vi "Climb Controller.vi"(8 "error in":errorcluster) -> ()   [LabVIEW 2020]
doc: "This VI executes continuously carrying out the current operation and responding to updates or new operations. It will often contain the timing or control code that is difficult to place directly in TeleOp. This VI generally opens all sensors and motors and isolates the rest of the robot code from knowing how the operations are carried out."
uses:
  <vilib>/Rock Robotics/WPI/Framework/Completion Status.ctl
  Climb Setpoints.ctl
  Climb Operations.ctl
  <vilib>/Rock Robotics/WPI/ThirdParty/Phoenix-LabVIEW/Motor Controller/Controls/CTRE_Phoenix_MotorControl_ControlMode.ctl
  <vilib>/Rock Robotics/Network Tables/NT Write Number.vi
panel:
  in  "Interactive Values":T1
  out "Current\nCmd":string
  in  "Buttons":cluster{"Execute Cmd":bool, "Abort Cmd":bool}
  out "Command Timing":cluster{"Start Time (ms)":u32, "Iterations":i32}
  out "Status":T3
  # "Tip: It may be helpful to observe inputs and sensor values.\nYou may also want to display tuning or debugging controls."
  # "Interactive Command: You may fill in the settings for a command\nand schedule it with the Execute button. You can observe and abort\nany command while fine tuning the code for the controller."
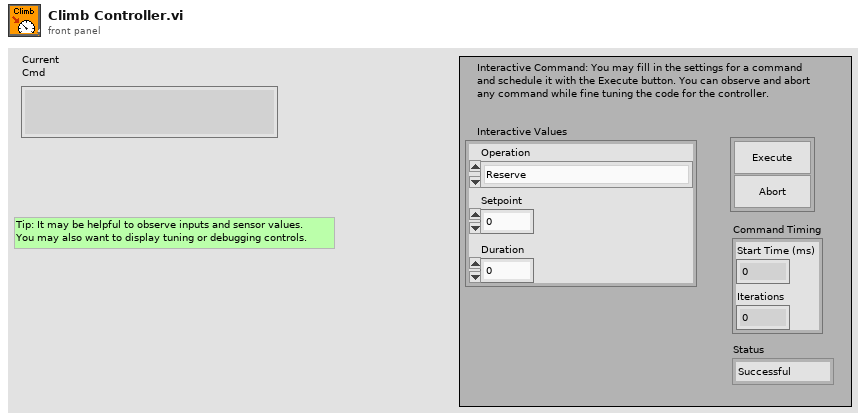
[diagram p1: front panel]
types:
  T1 = typedef "Climb Setpoints.ctl" = cluster{"Operation":T2, "Setpoint":dbl, "Duration":dbl}
  T2 = typedef "Climb Operations.ctl" = enum16{"Reserve", "Read Current", "Immediate", "Up", "Down"}
  T3 = typedef "Completion Status.ctl" = enum16{"Successful", "Aborted", "Incomplete"}
  T4 = typedef "WPI_MotorControlDeviceRef.ctl" = cluster{"DeviceStatus":errorcluster, "Type":T5, "PWM":cluster{"PWM Channel":T6, "DeadBand":T7}, "CAN":cluster{"Device Number":u8, "SetOutput VI Ref":variant, "GetOutput VI Ref":variant, "Enable VI Ref":variant, "Disable VI Ref":variant, "Data":variant}, "Invert":bool, "DIO PWM":cluster{"PWM \"Enable\" Channel":T6, "DIOChannel":T8, "PWM Rate":dbl}}
  T5 = typedef "WPI_MotorControlType.ctl" = enum16{"PWM", "CAN", "DIO PWM"}
  T6 = typedef "FPGA_DIOPWMChannel.ctl" = enum8{"PWM 0", "PWM 1", "PWM 2", "PWM 3", "PWM 4", "PWM 5", "PWM 6", "PWM 7", "PWM 8", "PWM 9", "PWM MXP 0", "PWM MXP 1", "PWM MXP 2", "PWM MXP 3", "PWM MXP 4", "PWM MXP 5", "PWM MXP 6", "PWM MXP 7", "PWM MXP 8", "PWM MXP 9", "Invalid"}
  T7 = typedef "WPI_PWMDeadband.ctl" = cluster{"Name":string, "maxPositivePwm":i32, "minPositivePwm":i32, "centerPwm":i32, "maxNegativePwm":i32, "minNegativePwm":i32, "angularRange":u16}
  T8 = typedef "FPGA_DIOChannel.ctl" = enum8{"DIO 0", "DIO 1", "DIO 2", "DIO 3", "DIO 4", "DIO 5", "DIO 6", "DIO 7", "DIO 8", "DIO 9", "DIO MXP 0", "DIO MXP 1", "DIO MXP 2", "DIO MXP 3", "DIO MXP 4", "DIO MXP 5", "DIO MXP 6", "DIO MXP 7", "DIO MXP 8", "DIO MXP 9", "DIO MXP 10", "DIO MXP 11", "DIO MXP 12", "DIO MXP 13", "DIO MXP 14", "DIO MXP 15", "SPI Port CS1", "SPI Port CS2", "SPI Port CS3", "SPI Port MISO", "SPI Port MOSI", "Invalid"}
  T9 = typedef "Command Status Info.ctl" = cluster{"Name":string, "Status":T3, "notifier out":T10}
  T10 = typedef "Completion Notifier.ctl" = refnum<notifier>
  T11 = cluster{"Current Command":T1, "Command Timing":cluster{"Start Time (ms)":u32, "Iterations":i32}, "Command Arguments":cluster{"Command Info":T9, "Description":string, "Default Command":T1, "queue out":refnum<queue>, "Subsystem Name":string}}
  T12 = typedef "CTRE_Phoenix_MotorControl_ControlMode.ctl" = u16
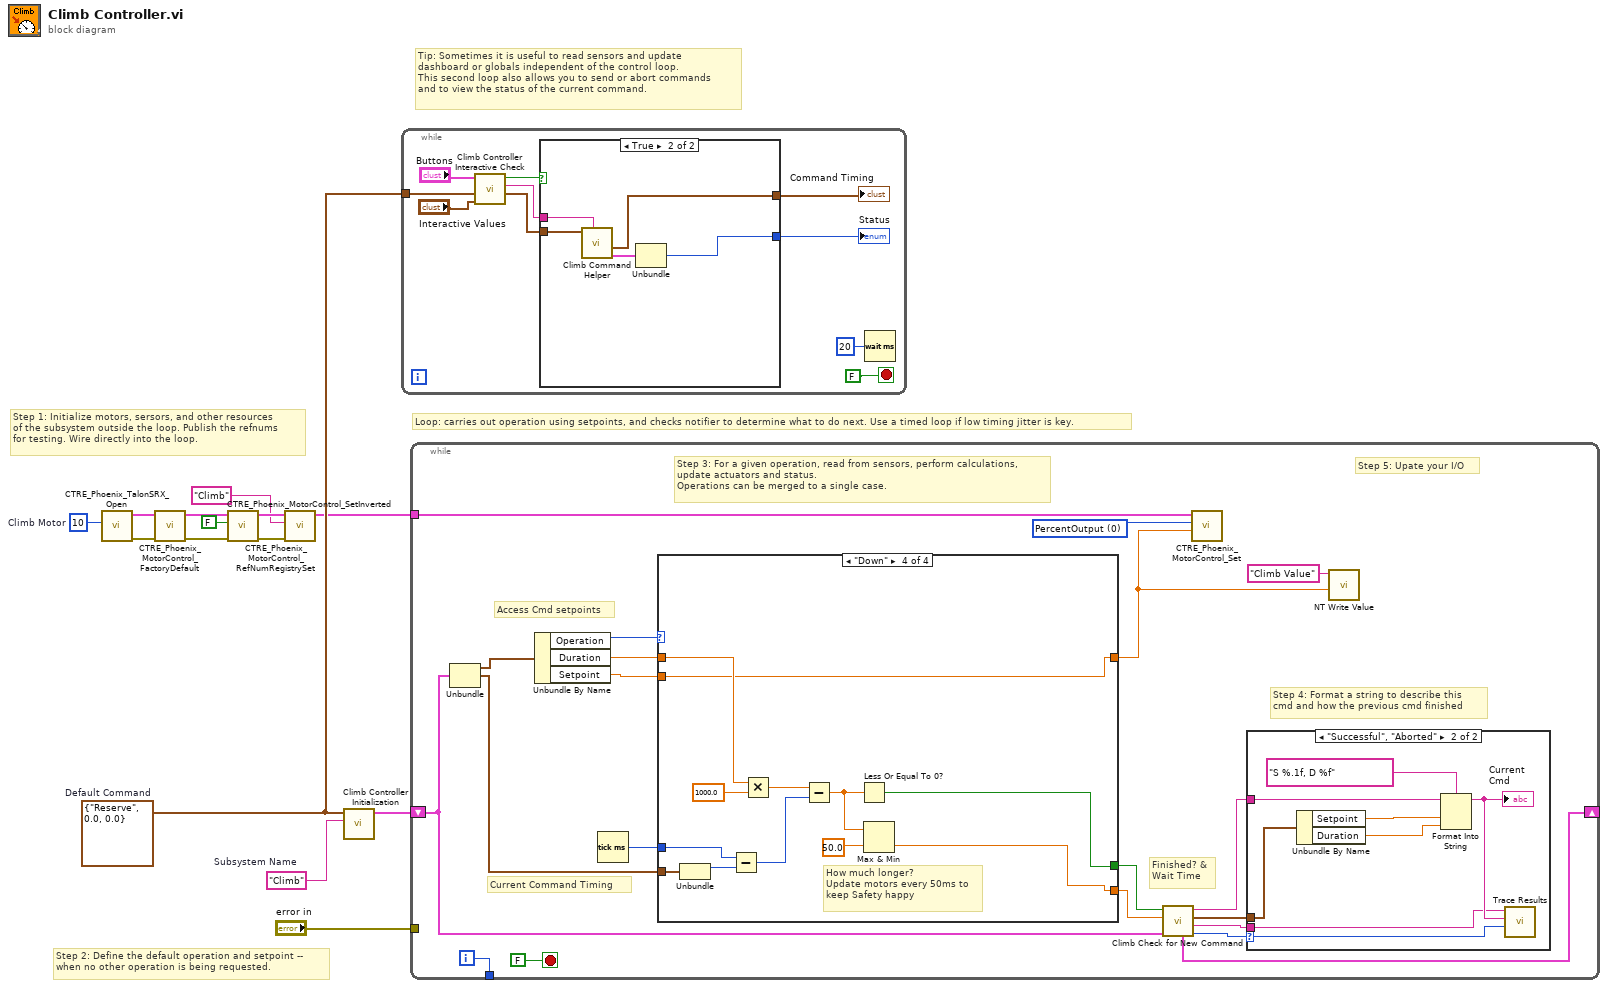
[diagram p0: block diagram]
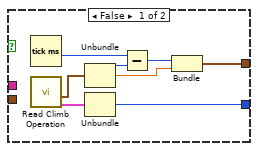
[diagram p2: hidden frame]
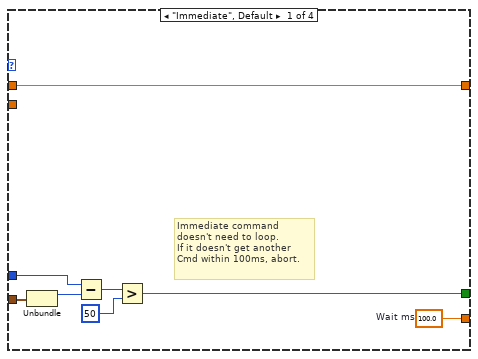
[diagram p4: hidden frame]
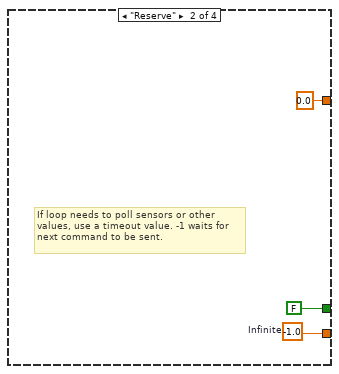
[diagram p5: hidden frame]
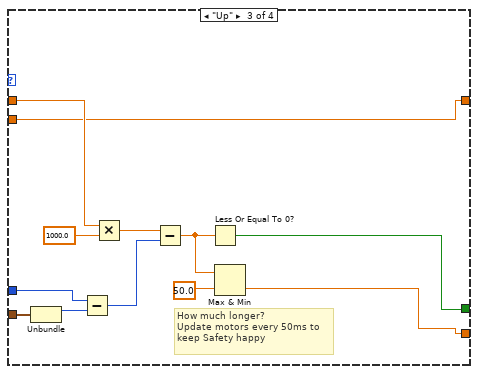
[diagram p6: hidden frame]
diagram:
  w2 = u8 10  # Climb Motor
  w11 = T1 {"Operation"=enum."Reserve", "Setpoint"=0.0, "Duration"=0.0}  # Default Command
  w12 = "Climb"  # Subsystem Name
  # "Tip: Sometimes it is useful to read sensors and update\ndashboard or globals independent of the control loop.\nThis second loop also allows you to send or abort commands\nand to view the status of the current command."
  # "Step 2: Define the default operation and setpoint --\nwhen no other operation is being requested."
  # "Step 1: Initialize motors, sersors, and other resources\nof the subsystem outside the loop. Publish the refnums\nfor testing. Wire directly into the loop."
  # "Loop: carries out operation using setpoints, and checks notifier to determine what to do next. Use a timed loop if low timing jitter is key."
  n1 = call <vilib>:"CTRE_Phoenix_TalonSRX_Open.vi"("Device Number"=w2) -> ("error out"=w10:errorcluster, "PhoenixMotorControlDevRef"=w9:T4)  [unwired: 9 in]
  n2 = call <vilib>:"CTRE_Phoenix_MotorControl_FactoryDefault.vi"("error in"=w10, "PhoenixMotorControlDevRef"=w9) -> ("error out"=w8:errorcluster, "PhoenixMotorControlDevRef"=w7:T4)  [unwired: 8 in]
  n3 = call <vilib>:"CTRE_Phoenix_MotorControl_SetInverted.vi"("error in (no error)"=w8, "Invert?"=FALSE, "PhoenixMotorControlDevRef"=w7) -> ("error out"=w6:errorcluster, "PhoenixMotorControlDevRef"=w5:T4)  [unwired: 7 in]
  n4 = call <vilib>:"CTRE_Phoenix_MotorControl_RefNumRegistrySet.vi"("error in (no error)"=w6, "refnum name"="Climb", "PhoenixMotorControlDevRef"=w5) -> ("PhoenixMotorControlDevRef"=w1:T4)  [unwired: 7 in, 1 out]
  n5 = call "Climb Controller Initialization.vi"("Subsystem Name"=w12, "Default Command"=w11) -> ("Current Command"=w13:T11)  [unwired: 9 in]
  n6 = while {
    tunnel: w11 -> [w21]
    stop <- FALSE stop-if-true
    n7 = call "Climb Controller Interactive Check.vi"("Interactive Command in"="Interactive Values", "Default Command"=w21, "Buttons"="Buttons") -> ("Interactive Command out"=w18:T1, "Trace String"=w19:string, "Schedule"=w20:bool)  [unwired: 6 in]
    n8 = case shown="True" w20 {
      tunnel: [w32 w37] -> w17
      tunnel: w18 -> [_ w35]
      tunnel: [w28 w33] -> w16
      tunnel: w19 -> [_ w36]
      frame False {
        n9 = Tick Count (ms)() -> (millisecond timer value=w27:u32)
        n10 = call "Read Climb Operation.vi"() -> ("Command Info"=w25:T9, "SubSystem Data"=w26:T1)  [unwired: 9 in, 1 out]
        n11 = Unbundle(w26) -> ("Operation"=w31:T2, "Setpoint"=w29:dbl)  [unwired: 1 out]
        n12 = Unbundle(w25) -> ("Status"=w32:T3)  [unwired: 2 out]
        n13 = Subtract(x=w27, y=w31) -> (x-y=w30:u32)
        n14 = Bundle(w30, "Setpoint"=w29) -> (w28:cluster{u32, "Setpoint":dbl})  [unwired: 1 in]
      }
      frame True {
        n15 = call "Climb Command Helper.vi"("Description"=w36, "SubSystem Data"=w35) -> ("Command Info Out"=w34:T9, "Command Timing"=w33:cluster{"Start Time (ms)":u32, "Iterations":i32})  [unwired: 7 in, 1 out]
        n16 = Unbundle(w34) -> ("Status"=w37:T3)  [unwired: 2 out]
      }
    }
    "Status" <- w17
    "Command Timing" <- w16
    n17 = Wait (ms)(milliseconds to wait=u32 20) -> ()  [unwired: 1 out]
  }
  n18 = while {
    shift-right: [w49] -> _
    shift-left: w13 -> [w42]
    tunnel: [w56] -> _
    tunnel: "error in" -> [_]
    tunnel: w1 -> [w41]
    i -> [w56]
    stop <- FALSE stop-if-true
    w40 = T12 0 items=["PercentOutput"=0, "Position"=1, "Velocity"=2, "Current"=3, "Follower"=5, "MotionProfile"=6, "MotionMagic"=7, "MotionProfileArc"=10, "Disabled"=15] ("Control Mode")
    # "Step 5: Upate your I/O"
    # "Step 4: Format a string to describe this\ncmd and how the previous cmd finished"
    # "Current Command Timing"
    # "Access Cmd setpoints"
    # "Finished? &\nWait Time"
    # "Step 3: For a given operation, read from sensors, perform calculations,\nupdate actuators and status.\nOperations can be merged to a single case."
    n19 = Unbundle(w42) -> ("Current Command"=w55:T1, "Command Timing"=w51:cluster{"Start Time (ms)":u32, "Iterations":i32})  [unwired: 1 out]
    n20 = Unbundle By Name(w55) -> ("Operation"=w54:T2, "Duration"=w53:dbl, "Setpoint"=w50:dbl)
    n21 = Tick Count (ms)() -> (millisecond timer value=w52:u32)
    n22 = case shown="\"Down\"" w54 {
      tunnel: [w73 w76 w79 w91] -> w47
      tunnel: [w67 FALSE ("ignore previous (F)") w80 w92] -> w48
      tunnel: w51 -> [w69 _ w82 w94]
      tunnel: w53 -> [w66 _ w78 w90]
      tunnel: w52 -> [w68 _ w81 w93]
      tunnel: w50 -> [_ _ w77 w89]
      tunnel: [w66 0.0 ("Duration") w77 w89] -> w39
      frame "Immediate", Default {
        w73 = 100.0  # Wait ms
        # "Immediate command\ndoesn't need to loop.\nIf it doesn't get another\nCmd within 100ms, abort."
        n23 = Unbundle(w69) -> ("Start Time (ms)"=w72:u32)  [unwired: 1 out]
        n24 = Subtract(x=w68, y=w72) -> (x-y=w71:u32)
        n25 = Greater?(x=w71, y=u8 50 ("Left Motor")) -> (0:w67:bool)
      }
      frame "Reserve" {
        w76 = -1.0  # Infinite
        # "If loop needs to poll sensors or other\nvalues, use a timeout value. -1 waits for\nnext command to be sent."
      }
      frame "Up" {
        # "How much longer?\nUpdate motors every 50ms to\nkeep Safety happy"
        n26 = Unbundle(w82) -> ("Start Time (ms)"=w85:u32)  [unwired: 1 out]
        n27 = Subtract(x=w81, y=w85) -> (x-y=w88:u32)
        n28 = Multiply(x=w78, y=1000.0) -> (x*y=w87:dbl)
        n29 = Subtract(x=w87, y=w88) -> (x-y=w84:dbl)
        n30 = Less Or Equal To 0?(x=w84) -> (x <= 0?=w80:bool)
        n31 = Max & Min(x=w84, y=50.0) -> (min(x,y)=w79:dbl)  [unwired: 1 out]
      }
      frame "Down" {
        # "How much longer?\nUpdate motors every 50ms to\nkeep Safety happy"
        n32 = Unbundle(w94) -> ("Start Time (ms)"=w97:u32)  [unwired: 1 out]
        n33 = Subtract(x=w93, y=w97) -> (x-y=w100:u32)
        n34 = Multiply(x=w90, y=1000.0) -> (x*y=w99:dbl)
        n35 = Subtract(x=w99, y=w100) -> (x-y=w96:dbl)
        n36 = Less Or Equal To 0?(x=w96) -> (x <= 0?=w92:bool)
        n37 = Max & Min(x=w96, y=50.0) -> (min(x,y)=w91:dbl)  [unwired: 1 out]
      }
    }
    n38 = call "Climb Check for New Command.vi"("Current Command"=w42, "Wait time (ms)"=w47, "Finished?"=w48) -> ("Completion"=w43:T3, "Subsystem Name"=w44:string, "Current Command"=w45:T1, "Initial Trace String"=w46:string, "NextCommand"=w49:T11)  [unwired: 4 in]
    n39 = call <vilib>:"CTRE_Phoenix_MotorControl_Set.vi"("Output"=w39, "Control Mode"=w40, "PhoenixMotorControlDevRef"=w41) -> ()  [unwired: 7 in, 2 out]
    n40 = case shown="\"Successful\", \"Aborted\"" w43 {
      selector: w43 -> [_ w65]
      tunnel: w46 -> [_ w61]
      tunnel: w45 -> [_ w62]
      tunnel: w44 -> [_ w58]
      frame "Incomplete", Default {
        # "Continuing current command"
      }
      frame "Successful", "Aborted" {
        # "Report and setup for next command"
        n41 = Unbundle By Name(w62) -> ("Setpoint"=w64:dbl, "Duration"=w59:dbl)
        n42 = Format Into String(format string="S %.1f, D %f", initial string=w61, w64, w59) -> (resulting string=w60:string)  [unwired: 1 in, 1 out]
        "Current\nCmd" <- w60
        n43 = call <vilib>:"Trace Results.vi"("Status of previous command"=w65, "Description"=w60, "Subsystem"=w58) -> ()  [unwired: 9 in]
      }
    }
    n44 = call-poly <vilib>:"NT Write Value.vi"("Numeric"=w39, "Name"="Climb Value") -> ()  [unwired: 9 in, 1 out]
  }
